vi "_Set Token.vi"(8 "error in (no error)":errorcluster, 10 "EventToken":refnum<class "EventToken.lvclass">, 11 "Event in":refnum<class "Event.lvclass">) -> (0 "error out":errorcluster, 3 "Event out":refnum<class "Event.lvclass">)   [LabVIEW 2021, in "EventManagerLibrary.lvlib" / "Event.lvclass"]
uses:
  Event.lvclass
  EventToken/EventToken.lvclass
  Event.lvclass/Event.ctl
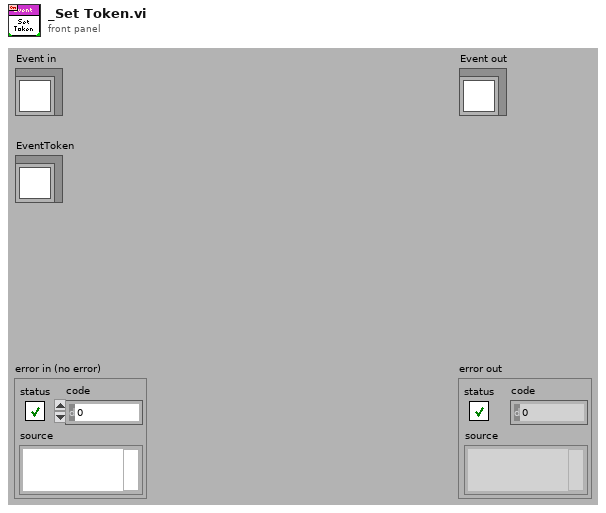
[diagram p1: front panel]
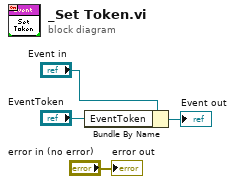
[diagram p0: block diagram]
diagram:
  n1 = Bundle By Name(cluster="Event in", "EventToken"="EventToken") -> (→"Event out":refnum<class "Event.lvclass">)
  "error out" <- "error in (no error)"
